vi "MainGui.vi"() -> ()   [LabVIEW 2016]
uses:
  MainGui.TopBar.ctl
  Tools/TouchPanel/TouchPanel.Keyboard.ctl
  Tools/EventLog/EventLog.Gui.Sets.ctl
  Tools/EventLog/EventLog.EventLevelOperatorGui.ctl
  Drivers/PLC/PLC.CheckStatusReassembly.ctl
  MainGui.Action.ctl
  <vilib>/Utility/miscctls.llb/LVRowAndColumnTypeDef.ctl
  <vilib>/Utility/miscctls.llb/LVRowAndColumnUnsignedTypeDef.ctl
  MainGui.UserMsg.ctl
  Tools/Translator/Translator.Message.ctl
  Tools/User/User.Level.ctl
  Tools/CitTemplate/citTemplate.errData.ctl
  Tools/EventLog/EventLog.EventSource.ctl
  Drivers/PLC/PLC.State.ctl
  Database/Database.Gui.ctl
  Database/Database.Gui.SingleTestValue.ctl
  Tools/Translator/Translator.FormatMessage.vi
  Tools/Config/Config.Global.vi
  Global/ApplicationGlobal.vi
  Drivers/PLC/PLC.Global.vi
  Tools/Translator/Translator.Global.vi
  <vilib>/Utility/inputDevices.llb/closeMouse.vi
  Tools/User/User.Global.vi
  Database/Database.Global.vi
panel:
  out "LastPlcRequest":T1
  out "LastRequestedProduct":cluster{"Variant":string, "Serial":string}
  out "RefreshDelay":timestamp
  in  "MainTab":enum32{"Monitor", "Logs"}(tab)
  in  "TESTER":bool
  in  "op30_2":bool caption="OP30_2"
  in  "op40":bool caption="OP40"
  in  "op30_1":bool caption="OP30_1"
  in  "op20":bool caption="OP20"
  in  "op10":bool caption="OP10"
  in  "check":bool
  in  "Serial":string
  in  "RefNum":string
  in  "StatusTable":i32(listbox)=-1
  in  "LogsMode":enum16{"Live", "Arch"}(ring) caption="Mode"
  in  "LogsOptions":T2 caption="Event.Sets" {"Source" items=["All", "Gui", "Cache", "PLC1", "PLC2", "PLC3", "DB", "DB01", "DB02", "DB03", "DB04", "DB05", "DB06", "DB07", "DB08", "DB09", "DB10", "DB11", "DB12", "DB13", "DB14", "DB15", "DB16"]; "Level" items=["ALL", "Debug", "Info", "Warning", "Error"]; "dtm_End" format="%<%.1X\n%x>T"; "dtm_Begin" format="%<%.1X\n%x>T"}
  out "LogsTable":i32(listbox)
  in  "Btn_Exit":bool
  in  "Btin_LogIn":bool
  in  "Btn_Monitor":bool
  in  "TopBar":T4={"_loop"=4, "time"="", "~flag"=bytes[0], "~touchpanel"=FALSE, "ver"="", "~msg"="", "DB"=0, "PLC"=0} {"PLC" items=["OK", "ALL", "PLC01"]; "DB" items=["OK", "ALL", "ST01"]}
  in  "start here":bool
  out "StatusMsg":string
  out "DeviceID":refnum<k1> caption="device ID"
  in  "Btn_ErrConfirm":bool
  out "ErrMsg":i32(listbox)
  in  "Btn_Logs":bool
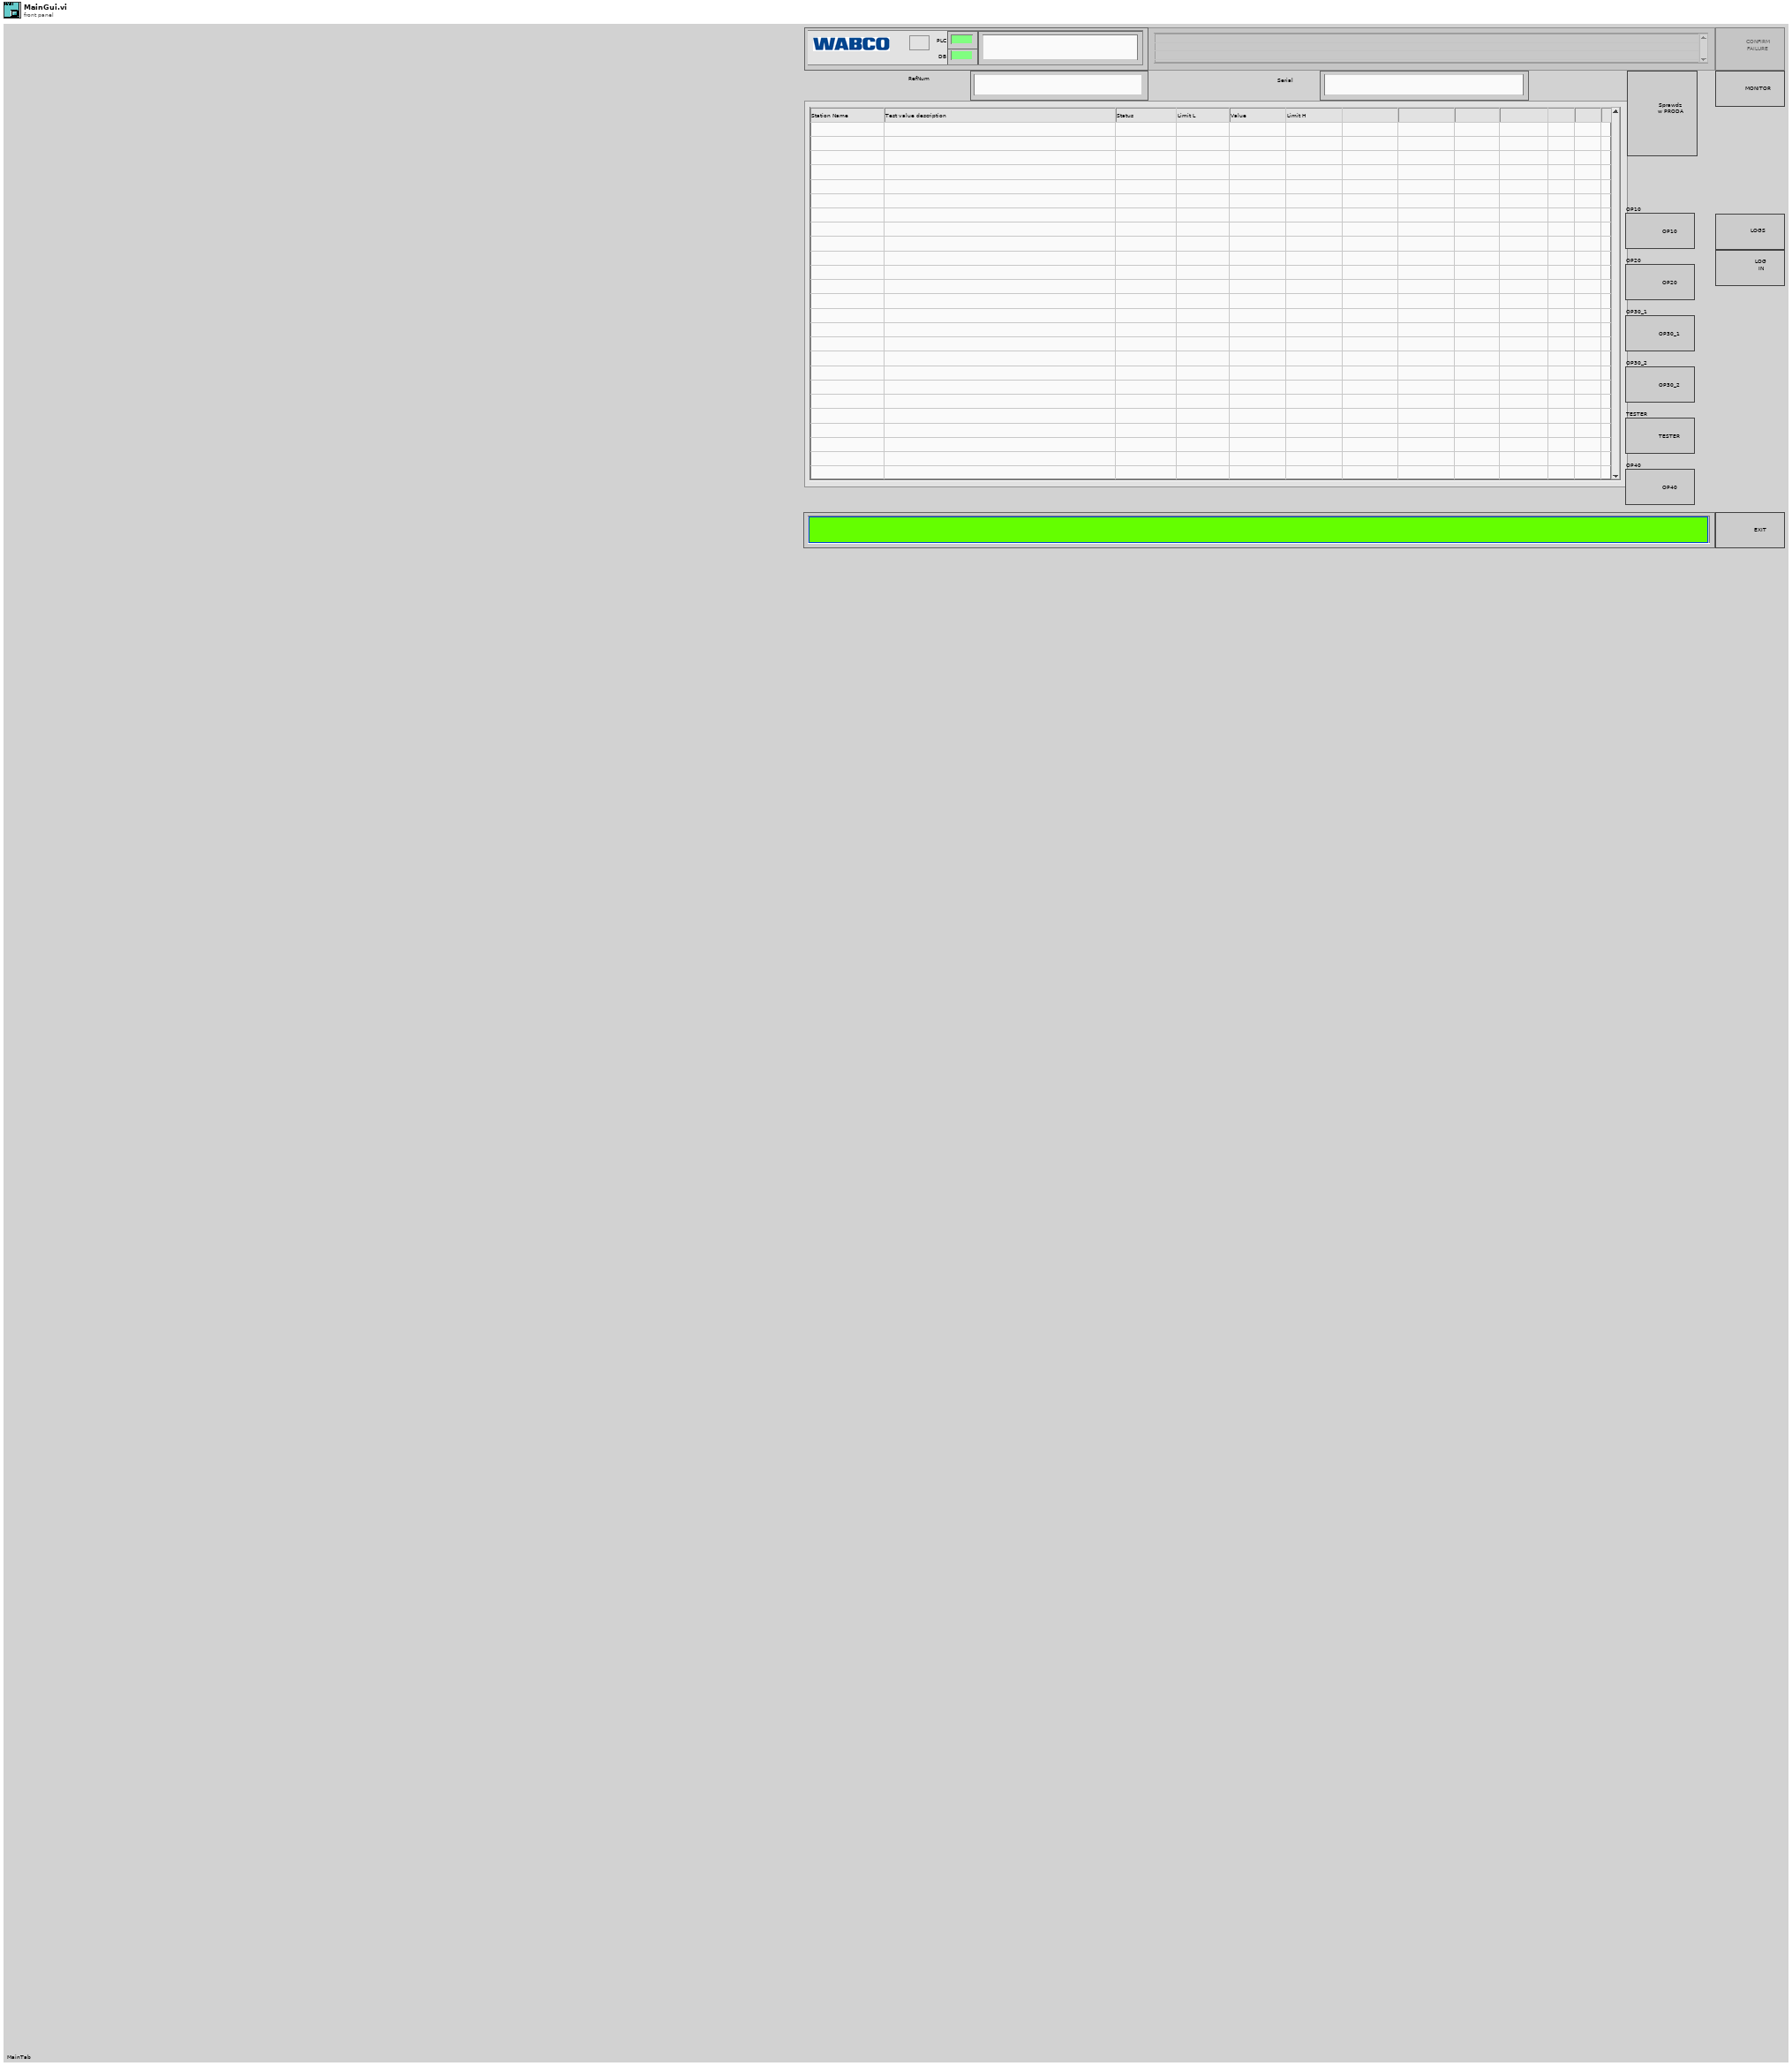
[diagram p1: front panel]
types:
  T1 = typedef "PLC.CheckStatusReassembly.ctl" = cluster{"Ref":string, "Serial":string, "Station":string}
  T2 = typedef "EventLog.Gui.Sets.ctl" = cluster{"IncludeBegin":bool, "dtm_Begin":timestamp, "IncludeEnd":bool, "dtm_End":timestamp, "Events Level Operator":T3, "Level":u16, "Source":u16, "SearchText":string, "Refresh":bool, "Pages":i32, "PageNo":i32, "First":bool, "Prev":bool, "Next":bool, "Last":bool}
  T3 = typedef "EventLog.EventLevelOperatorGui.ctl" = enum16{">=", "=", "<="}
  T4 = typedef "MainGui.TopBar.ctl" = cluster{"_loop":i32, "time":string, "~flag":picture, "~touchpanel":T5, "ver":string, "~msg":string, "DB":u16, "PLC":u16}
  T5 = typedef "TouchPanel.Keyboard.ctl" = bool
  T6 = typedef "Translator.Message.ctl" = enum16{"-", "Event confirmed", "Log out", "Log in", "Shutdown", "Cancel", "Start", "Continue", "Stop", "On", "Off", "OK", "NOK", "NOK %s", "This", "Prev", "Home", "Work", "In progress...", "Missing", "Empty", "Hardware failure", "Initial", "Error %d >> %s", "Error %d >> %s >> %s", "Starting %s", "Quitting %s", "Configured", "Initializing", "Quitting", "Loading", "Running %s", "Stopped", "Summary", "Do you want to continue?", "Do you want to exit?", "Log out?", "System", "All", "IDLE", "Translating...%s", "Not found", "Alarm %s", "Run", "Skip", "Abort", "Repeat", "Please wait...", "Database disconnected", "Login to database successful", "Login to database failed: %d; %s", "Get process step data for %s", "Changeover off", "Changeover into %s", "Product %s | %s found in cache with status %d at previous station", "Product %s | %s found in database with status %d at previous station", "Product %s | %s not found in cache at previous station", "Product %s | %s not found in database at previous station", "Product %s | %s found in cache with status %d at this station (%d repetion)", "Product %s | %s found in database with status %d at this station (%d repetition)", "Product %s | %s not found in cache at this station", "Product %s | %s not found in database at this station", "Product %s | %s found in cache for component %s | %s", "Product %s | %s found in database for component %s | %s", "Product not found in cache for component %s | %s", "Product not found in database for component %s | %s", "Product %s | %s connected with component %s | %s (cache)", "Product %s | %s connected with component %s | %s (database)", "New data for %s | %s (cache)", "New data for %s | %s (database)", "File %s moved (cache)", "File %s deleted (cache)", "Msg %d >> %s", "PLC LifeBit Failure", "Reconnecting DB", "Reconnecting PLC", "Free disk space is below 1GB - contact technician", "Unable to check product status", "Product %s SN %s checked in DB", "Unable To check status from station %s"}
  T7 = enum8{"Enabled", "Disabled", "Disabled and Grayed Out"}
  T8 = typedef "LVRowAndColumnUnsignedTypeDef.ctl" = cluster{"Row":u32, "Column":u32}
  T9 = typedef "LVRowAndColumnTypeDef.ctl" = cluster{"Row":i32, "Column":i32}
  T10 = enum32{"invalid app kind", "Development System", "Run Time System", "Student Edition", "Embedded LabVIEW", "Evaluation", "Custom"}
  T11 = enum32{"Invalid", "Standard", "Closed", "Hidden", "Minimized", "Maximized"}
  T12 = typedef "MainGui.UserMsg.ctl" = cluster{"Msg":T6, "Arguments":variant[], "BgColor":u32, "TxtColor":u32, "Blink":bool}
  T13 = typedef "User.Level.ctl" = enum16{"-", "Operator", "Technician", "Administrator"}
  T14 = typedef "citTemplate.errData.ctl" = cluster{"ts":timestamp, "src":T15, "instance":i32, "action":string, "error":errorcluster, "unconfirmed":bool}
  T15 = typedef "EventLog.EventSource.ctl" = enum16{"All", "Gui", "Cache", "PLC1", "PLC2", "PLC3", "DB", "DB01", "DB02", "DB03", "DB04", "DB05", "DB06", "DB07", "DB08", "DB09", "DB10", "DB11", "DB12", "DB13", "DB14", "DB15", "DB16"}
  T16 = typedef "PLC.State.ctl" = enum32{"Off", "Error", "Idle", "Run"}
  T17 = typedef "Database.Gui.ctl" = cluster{"Station":string, "ButtonEnabled":bool, "Values":T18[]}
  T18 = typedef "Database.Gui.SingleTestValue.ctl" = cluster{"EV_name":string, "Value":dbl, "LimitL":dbl, "LimitH":dbl, "Status":u8}
  T19 = typedef "MainGui.Action.ctl" = enum32{"idle", "constructor", "destructor", "--- MainGui ---", "Gui.Translate", "Error.Update", "Error.Confirm", "TopBar.Update", "Buttons.Update", "StatusMsg.Update", "StatusTable.Update", "LogsTable.Update", "PLCReasemblyDone"}
  T20 = typedef "LVPositionTypeDef.ctl" = cluster{"Left":i32, "Top":i32}
  T21 = typedef "PLC.Data.Status.ctl" = cluster{"Idx":i32, "ConnRef":u64, "State":T16, "LiveBitTimer":timestamp}
  T22 = typedef "Database.Handler.Data.Status.ctl" = cluster{"Run":bool, "Handle":i32, "ConnTS":timestamp, "DbTime":timestamp, "DbTimeOffset":dbl}
  T23 = typedef "Database.Data.Sets.ctl" = cluster{"Enable":bool, "ConnString":string, "SystemName":string, "Process.Begin":bool, "Process.End":bool}
  T24 = typedef "PLC.Data.Sets.ctl" = cluster{"Enable":bool, "IP":string, "Rack":i32, "Slot":i32, "LifeBitTimer_s":dbl, "DataBlockAddr_PCStatus":i32, "DataBlockAddr_PLCStatus":i32, "DataBlockAddr_PLCNewData":i32[], "DataBlockSize_PLCNewData":i32[], "DataBlockAddr_PLCChangeOver":i32[], "DataBlockSize_PLCChangeOver":i32[], "DataBlockAddr_PCChangeOver":i32[], "DataBlockAddr_PLCCheckStatus":i32[], "DataBlockSize_PLCCheckStatus":i32[], "DataBlockAddr_PCCheckStatus":i32[]}
  T25 = typedef "EventLog.EventGui.ctl" = cluster{"ts":dbl, "lev":T26, "src":T15, "msg":T6, "arg":variant[], "msg_str":string}
  T26 = typedef "EventLog.EventLevel.ctl" = enum8{"Debug", "Info", "Warning", "Error"}
  T27 = cluster{"Ref":bool, "Serial":bool, "Station":bool}
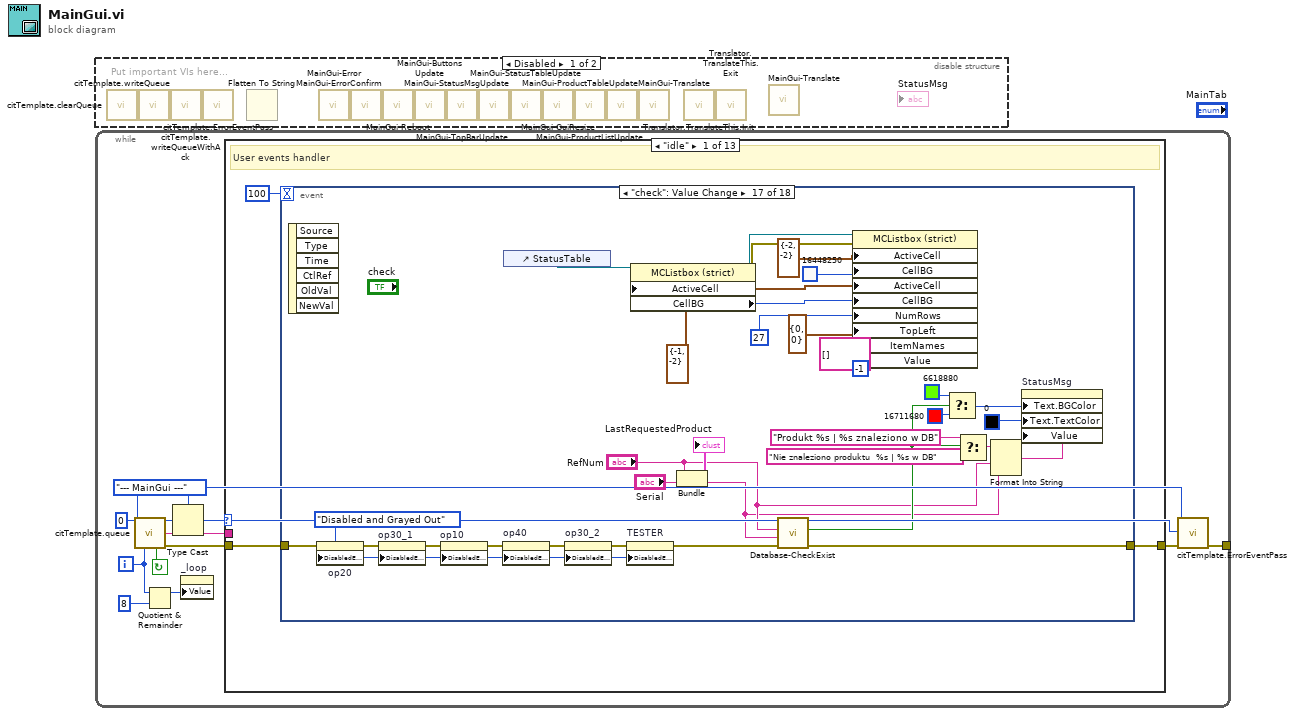
[diagram p0: block diagram]
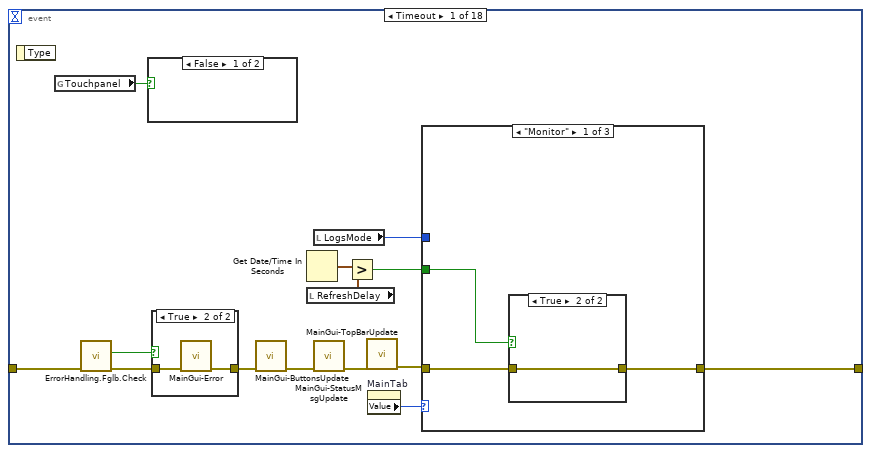
[diagram p3: hidden frame]
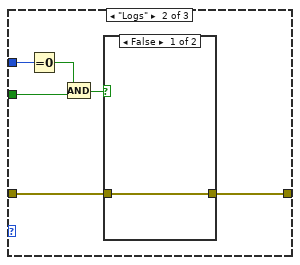
[diagram p6: hidden frame]
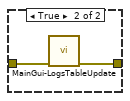
[diagram p7: hidden frame]
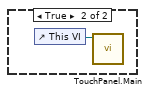
[diagram p9: hidden frame]
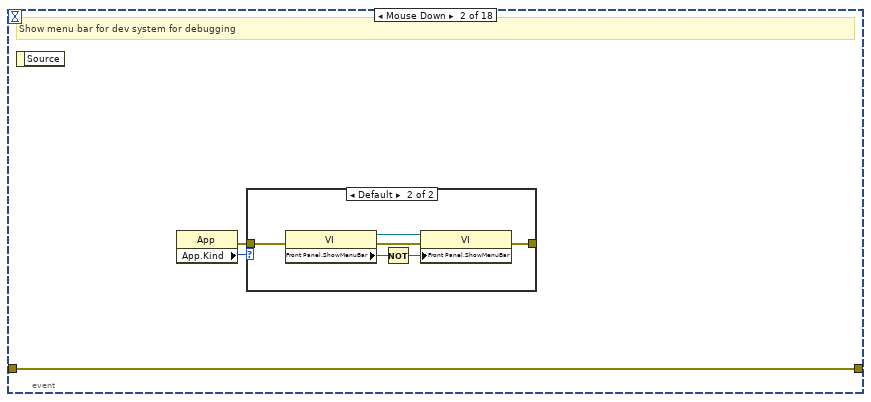
[diagram p10: hidden frame]
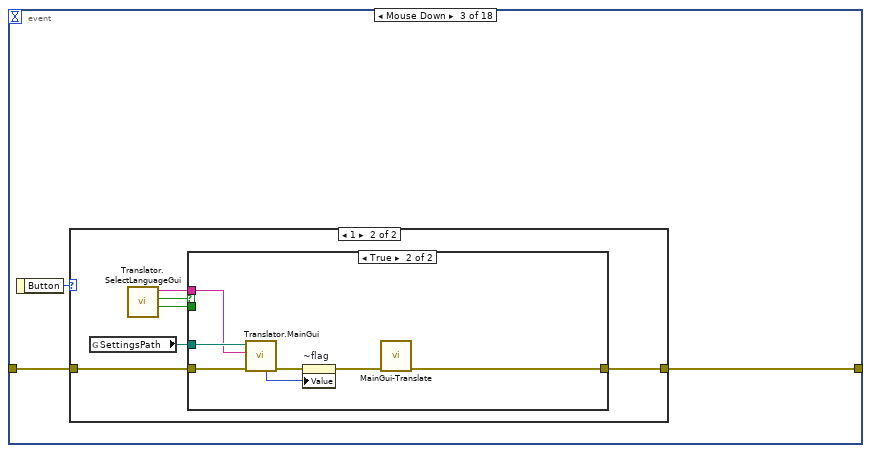
[diagram p12: hidden frame]
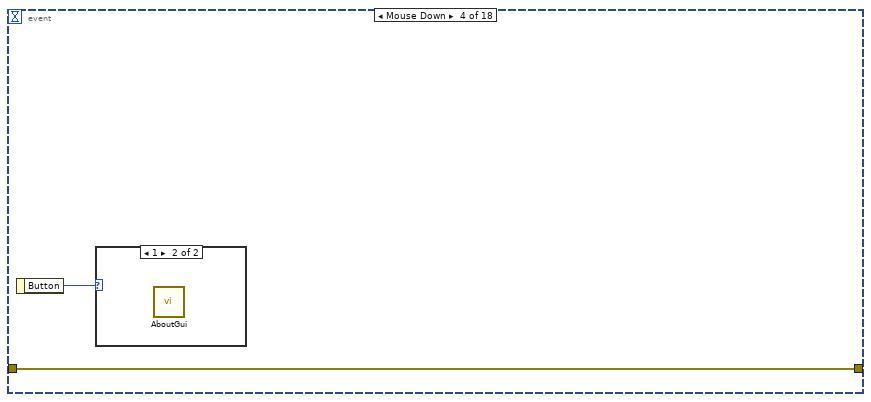
[diagram p15: hidden frame]
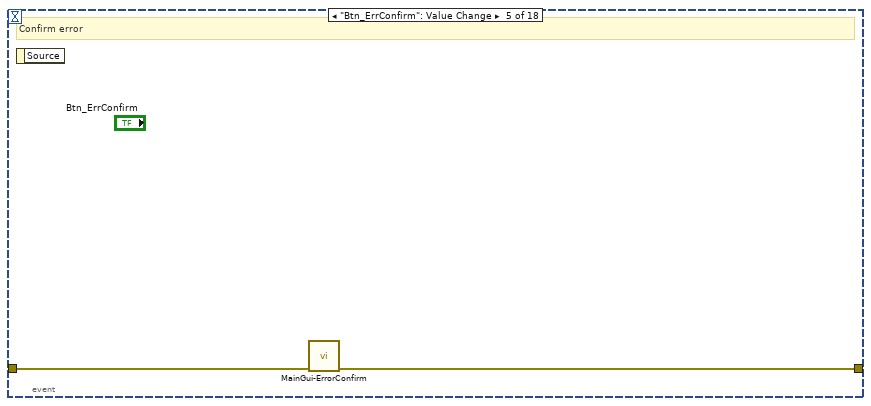
[diagram p17: hidden frame]
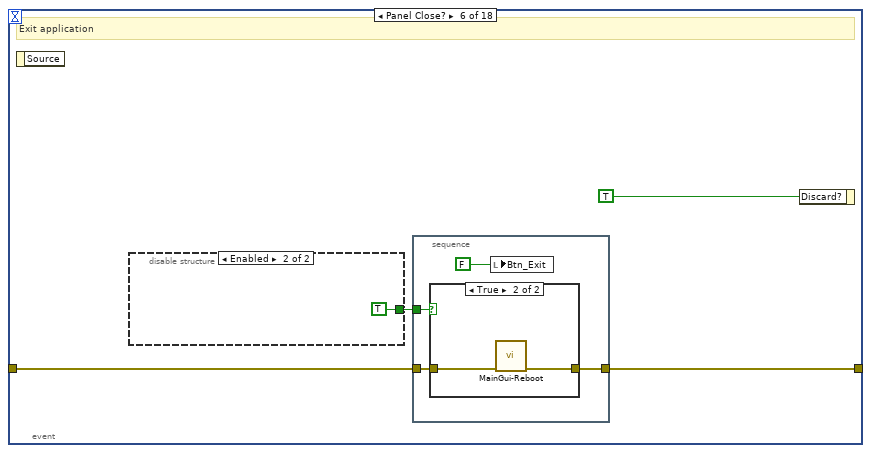
[diagram p18: hidden frame]
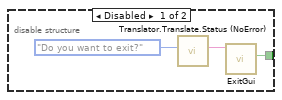
[diagram p19: hidden frame]
diagram:
  n1 = disable-structure shown="Disabled" {
    frame Disabled {
      # "Put important VIs here..."
      n2 = call "citTemplate.clearQueue.vi"() -> ()  [unwired: 14 in, 2 out]
      n3 = call "citTemplate.writeQueue.vi"() -> ()  [unwired: 15 in, 1 out]
      n4 = call "citTemplate.writeQueueWithAck.vi"() -> ()  [unwired: 13 in, 3 out]
      n5 = call "citTemplate.ErrorEventPass.vi"() -> ()  [unwired: 11 in, 1 out]
      n6 = Flatten To String() -> ()  [unwired: 4 in, 3 out]
      n7 = call "MainGui-Error.vi"() -> ()  [unwired: 11 in, 1 out]
      n8 = call "MainGui-ErrorConfirm.vi"() -> ()  [unwired: 11 in, 1 out]
      n9 = call "MainGui-Reboot.vi"() -> ()  [unwired: 11 in, 1 out]
      n10 = call "MainGui-ButtonsUpdate.vi"() -> ()  [unwired: 11 in, 1 out]
      n11 = call "MainGui-TopBarUpdate.vi"() -> ()  [unwired: 11 in, 1 out]
      n12 = call "MainGui-StatusMsgUpdate.vi"() -> ()  [unwired: 11 in, 1 out]
      n13 = call "MainGui-StatusTableUpdate.vi"() -> ()  [unwired: 11 in, 1 out]
      n14 = call "MainGui-GuiResize.vi"() -> ()  [unwired: 11 in, 1 out]
      n15 = call "MainGui-ProductListUpdate.vi"() -> ()  [unwired: 11 in, 1 out]
      n16 = call "MainGui-ProductTableUpdate.vi"() -> ()  [unwired: 11 in, 1 out]
      n17 = call "MainGui-Translate.vi"() -> ()  [unwired: 11 in, 1 out]
      n18 = call "Translator.TranslateThis.Init.vi"() -> ()  [unwired: 11 in, 1 out]
      n19 = call "Translator.TranslateThis.Exit.vi"() -> ()  [unwired: 11 in, 1 out]
      n20 = call "MainGui-Translate.vi"() -> ()  [unwired: 11 in, 1 out]
    }
    frame Enabled {
    }
  }
  n21 = while {
    tunnel: [w5] -> _
    i -> [w6]
    stop <- w9 continue-if-true
    w8 = MainGui.Action."--- MainGui ---" ("Action")
    n22 = call "citTemplate.queue.vi"("ms timeout (250 ms)"=0, "event enum"=w8, "iteration (-1)"=w6) -> ("event out"=w12:u32, "(flatten) data out"=w11:string, "continue"=w9:bool, "error out"=w10:errorcluster)  [unwired: 2 in, 7 out]
    n23 = Quotient & Remainder(x=w6, y=8) -> (x-y*floor(x/y)=w1:i32)  [unwired: 1 out]
    n24 = Type Cast(type=w8, x=w12) -> (*(type *) &x=w4:T19)
    n25 = property on="_loop" class="Ring (strict)"("Value"=w1) -> ()  [unwired: 2 in, 2 out]
    n26 = case shown="\"idle\"" w4 {
      tunnel: w11 -> [_ _ _ w315 _ _ _ _ _ _ w458 _ w568]
      tunnel: w10 -> [w15 w228 w285 w317 w319 w323 w360 w361 w409 w413 w460 w517 w587]
      tunnel: [w14 w227 w284 w314 w322 w324 w359 w361 w409 w412 w445 w516 w569] -> w2
      frame "idle" {
        # "User events handler"
        n27 = event shown="[16] \"check\": Value Change" {
          selector: _ -> [_ _ _ _ _ _ _ _ _ _ _ _ _ _ _ _ _ _]
          dyn-events: _ -> [_ _ _ _ _ _ _ _ _ _ _ _ _ _ _ _ _ _]
          timeout: 100 -> [_ _ _ _ _ _ _ _ _ _ _ _ _ _ _ _ _ _]
          tunnel: w15 -> [w25 w51 w60 w77 w80 w83 w98 w113 w119 w125 w128 w135 w140 w148 w156 w161 w180 w220]
          tunnel: [w26 w51 w59 w77 w79 w82 w97 w113 w119 w125 w127 w134 w140 w148 w156 w161 w193 w208] -> w14
          event Timeout {
            n28 = event-data() -> ()  [unwired: 1 in, 1 out]
            n29 = global read "Config.Global.vi" "Touchpanel"() -> (w29:bool)
            n30 = call "ErrorHandling.Fglb.Check.vi"("error in (no error)"=w25) -> ("error out"=w24:errorcluster, "changed?"=w23:bool)  [unwired: 9 in]
            n31 = case shown="False" w29 {
              frame False {
              }
              frame True {
                n32 = control-ref of="This VI"() -> (w48:refnum<vi>)
                n33 = call "TouchPanel.Main.vi"("VI ref"=w48) -> ()  [unwired: 9 in, 2 out]
              }
            }
            n34 = case shown="True" w23 {
              tunnel: [w30 w32] -> w28
              tunnel: w24 -> [w30 w31]
              frame False {
              }
              frame True {
                n35 = call "MainGui-Error.vi"("error in (no error)"=w31) -> ("error out"=w32:errorcluster)  [unwired: 10 in]
              }
            }
            n36 = call "MainGui-ButtonsUpdate.vi"("error in (no error)"=w28) -> ("error out"=w18:errorcluster)  [unwired: 10 in]
            n37 = Get Date/Time In Seconds() -> (seconds since 1Jan1904=w22:timestamp)
            n38 = local read "RefreshDelay"() -> (w21:timestamp)
            n39 = local read "LogsMode"() -> (w19:enum16{"Live", "Arch"})
            n40 = call "MainGui-StatusMsgUpdate.vi"("error in (no error)"=w18) -> ("error out"=w17:errorcluster)  [unwired: 10 in]
            n41 = Greater?(x=w22, y=w21) -> (0:w20:bool)
            n42 = call "MainGui-TopBarUpdate.vi"("error in (no error)"=w17) -> ("error out"=w16:errorcluster)  [unwired: 10 in]
            n43 = property on="MainTab" class="TabCtl (strict)"() -> ("Value"=w27:enum32{"Monitor", "Logs"})  [unwired: 2 in, 2 out]
            n44 = case shown="\"Monitor\"" w27 {
              tunnel: w16 -> [w35 w39 w47]
              tunnel: [w34 w38 w47] -> w26
              tunnel: w20 -> [w33 w42 _]
              tunnel: w19 -> [_ w43 _]
              frame "Monitor" {
                n45 = case shown="True" w33 {
                  tunnel: w35 -> [w36 w37]
                  tunnel: [w36 w37] -> w34
                  frame False {
                  }
                  frame True {
                  }
                }
              }
              frame "Logs" {
                n46 = Equal To 0?(x=w43) -> (x = 0?=w41:bool)
                n47 = Compound Arithmetic op=AND(w41, w42) -> (w40:bool)
                n48 = case shown="False" w40 {
                  tunnel: w39 -> [w44 w46]
                  tunnel: [w44 w45] -> w38
                  frame False {
                  }
                  frame True {
                    n49 = call "MainGui-LogsTableUpdate.vi"("error in (no error)"=w46) -> ("error out"=w45:errorcluster)  [unwired: 10 in]
                  }
                }
              }
              frame Default {
              }
            }
          }
          event Mouse Down {
            # "Show menu bar for dev system for debugging"
            n50 = event-data() -> ()  [unwired: 1 in, 1 out]
            n51 = property class="App"() -> (error out=w49:errorcluster, "App.Kind"=w50:T10)  [unwired: 2 in, 1 out]
            n52 = case shown="Default" w50 {
              tunnel: w49 -> [w52 w54]
              tunnel: [w52 w53] -> _
              frame "Run Time System" {
              }
              frame Default {
                n53 = property class="VI"(error in=w54) -> (reference out=w58:refnum<vi>, error out=w57:errorcluster, "Front Panel.ShowMenuBar"=w56:bool)  [unwired: 1 in]
                n54 = Not(x=w56) -> (.not. x?=w55:bool)
                n55 = property class="VI"(reference=w58, error in=w57, "Front Panel.ShowMenuBar"=w55) -> (error out=w53:errorcluster)  [unwired: 1 out]
              }
            }
          }
          event Mouse Down {
            n56 = event-data() -> ("Button"=w61:u16)  [unwired: 1 in]
            n57 = case shown="1" w61 {
              tunnel: w60 -> [w62 w66]
              tunnel: [w62 w65] -> w59
              frame Default {
              }
              frame 1 {
                n58 = global read "ApplicationGlobal.vi" "SettingsPath"() -> (w63:path)
                n59 = call "Translator.SelectLanguageGui.vi"() -> ("english"=w67:bool, "changed"=w68:bool, "Language"=w64:string)  [unwired: 9 in]
                n60 = case shown="True" w68 {
                  tunnel: w67 -> [_ _]
                  tunnel: w66 -> [w69 w76]
                  tunnel: [w69 w70] -> w65
                  tunnel: w64 -> [_ w74]
                  tunnel: w63 -> [_ w75]
                  frame False {
                  }
                  frame True {
                    n61 = call "Translator.MainGui.vi"("~error in"=w76, "~Language in use"=w74, "~Translation folder"=w75) -> ("~error out"=w73:errorcluster, "~flag small"=w72:picture)  [unwired: 5 in, 2 out]
                    n62 = property on="~flag" class="Pict"(error in=w73, "Value"=w72) -> (error out=w71:errorcluster)  [unwired: 1 in, 1 out]
                    n63 = call "MainGui-Translate.vi"("error in (no error)"=w71) -> ("error out"=w70:errorcluster)  [unwired: 10 in]
                  }
                }
              }
            }
          }
          event Mouse Down {
            n64 = event-data() -> ("Button"=w78:u16)  [unwired: 1 in]
            n65 = case shown="1" w78 {
              frame Default {
              }
              frame 1 {
                n66 = call "AboutGui.vi"() -> ()  [unwired: 12 in]
              }
            }
          }
          event "Btn_ErrConfirm": Value Change {
            # "Confirm error"
            n67 = event-data() -> ()  [unwired: 1 in, 1 out]
            n68 = call "MainGui-ErrorConfirm.vi"("error in (no error)"=w80) -> ("error out"=w79:errorcluster)  [unwired: 10 in]
          }
          event Panel Close? {
            # "Exit application"
            n69 = event-data() -> ()  [unwired: 1 in, 1 out]
            n70 = disable-structure shown="Enabled" {
              disable-tunnel: [w87 TRUE ("ok")] -> w84
              frame Disabled {
                n71 = call "Translator.Translate.Status (NoError).vi"("msg"=Translator.Message."Do you want to exit?") -> ("Translated Msg"=w85:string)  [unwired: 10 in]
                n72 = call "ExitGui.vi"("Message"=w85) -> ("ok"=w87:bool)  [unwired: 9 in, 1 out]
              }
              frame Enabled {
              }
            }
            n73 = stacked-sequence {
              tunnel: [w92] -> w82
              tunnel: w83 -> [w90]
              tunnel: w84 -> [w89]
              frame #0 {
                n74 = case shown="True" w89 {
                  tunnel: w90 -> [w93 w94]
                  tunnel: [w93 w95] -> w92
                  frame False {
                  }
                  frame True {
                    n75 = call "MainGui-Reboot.vi"("error in (no error)"=w94) -> ("error out"=w95:errorcluster)  [unwired: 10 in]
                  }
                }
                n76 = local write "Btn_Exit"(FALSE ("Btn_SelMode")) -> ()
              }
            }
            n77 = event-data("Discard?"=TRUE) -> ()  [unwired: 1 in, 1 out]
          }
          event "Btn_Exit": Value Change {
            # "Exit application"
            n78 = event-data() -> ()  [unwired: 1 in, 1 out]
            n79 = disable-structure shown="Disabled" {
              disable-tunnel: [w102 TRUE ("ok")] -> w99
              frame Disabled {
                n80 = call "Translator.Translate.Status (NoError).vi"("msg"=Translator.Message."Do you want to exit?") -> ("Translated Msg"=w100:string)  [unwired: 10 in]
                n81 = call "ExitGui.vi"("Message"=w100) -> ("ok"=w102:bool)  [unwired: 9 in, 1 out]
              }
              frame Enabled {
              }
            }
            n82 = property on="Btn_Exit" class="Bool (strict)"("Value"=FALSE ("Btn_Exit")) -> ()  [unwired: 2 in, 2 out]
            n83 = stacked-sequence {
              tunnel: [w106] -> w97
              tunnel: w98 -> [w105]
              tunnel: w99 -> [w104]
              frame #0 {
                n84 = case shown="True" w104 {
                  tunnel: w105 -> [w107 w108]
                  tunnel: [w107 w109] -> w106
                  frame False {
                  }
                  frame True {
                    n85 = call "MainGui-Reboot.vi"("error in (no error)"=w108) -> ("error out"=w109:errorcluster)  [unwired: 10 in]
                  }
                }
              }
            }
          }
          event "Btin_LogIn": Value Change {
            # "Log in/out"
            n86 = event-data() -> ()  [unwired: 1 in, 1 out]
            n87 = global write "ApplicationGlobal.vi" "Unlock"("Btin_LogIn") -> ()
            n88 = Select(t=T7."Enabled" ("Disabled"), s="Btin_LogIn", f=T7."Disabled and Grayed Out") -> ()  [unwired: 1 out]
          }
          event "Btn_Monitor": Value Change {
            w118 = TRUE ("Btn_Monitor")
            n89 = event-data() -> ()  [unwired: 1 in, 1 out]
            n90 = property on="MainTab" class="TabCtl (strict)"("Value"=0) -> ()  [unwired: 2 in, 2 out]
            n91 = property on="Btn_Monitor" class="Bool (strict)"("Value"=w118) -> (error out=w114:errorcluster)  [unwired: 2 in, 1 out]
            n92 = Not(x=w118) -> (.not. x?=w116:bool)
            n93 = Get Date/Time In Seconds() -> (seconds since 1Jan1904=w115:timestamp)
            n94 = local write "RefreshDelay"(w115) -> ()
            n95 = property on="Btn_Logs" class="Bool (strict)"(error in=w114, "Value"=w116) -> ()  [unwired: 1 in, 2 out]
          }
          event "Btn_Logs": Value Change {
            w124 = TRUE ("Btn_Monitor")
            n96 = event-data() -> ()  [unwired: 1 in, 1 out]
            n97 = property on="MainTab" class="TabCtl (strict)"("Value"=1) -> ()  [unwired: 2 in, 2 out]
            n98 = property on="Btn_Logs" class="Bool (strict)"("Value"=w124) -> (error out=w123:errorcluster)  [unwired: 2 in, 1 out]
            n99 = Not(x=w124) -> (.not. x?=w121:bool)
            n100 = property on="Btn_Monitor" class="Bool (strict)"(error in=w123, "Value"=w121) -> ()  [unwired: 1 in, 2 out]
            n101 = Get Date/Time In Seconds() -> (seconds since 1Jan1904=w120:timestamp)
            n102 = local write "RefreshDelay"(w120) -> ()
          }
          event "LogsMode": Value Change {
            n103 = event-data() -> ()  [unwired: 1 in, 1 out]
            n104 = Greater Than 0?(x="LogsMode") -> (x > 0?=w130:bool)
            n105 = Select(t=T7."Enabled" ("Disabled"), s=w130, f=T7."Disabled" ("Disabled")) -> (s? t:f=w126:T7)
            n106 = Not(x=w130) -> (.not. x?=w129:bool)
            n107 = property on="PageNo" class="DigNum (strict)"("DisabledEnum"=w126) -> ()  [unwired: 2 in, 2 out]
            n108 = property on="LogsTable" class="MCListbox (strict)"("HScrollVis"=w129) -> ()  [unwired: 2 in, 2 out]
            n109 = property on="First" class="Bool (strict)"("DisabledEnum"=w126) -> ()  [unwired: 2 in, 2 out]
            n110 = property on="Prev" class="Bool (strict)"("DisabledEnum"=w126) -> ()  [unwired: 2 in, 2 out]
            n111 = call "MainGui-LogsTableUpdate.vi"("error in (no error)"=w128) -> ("error out"=w127:errorcluster)  [unwired: 10 in]
            n112 = property on="Next" class="Bool (strict)"("DisabledEnum"=w126) -> ()  [unwired: 2 in, 2 out]
            n113 = property on="Last" class="Bool (strict)"("DisabledEnum"=w126) -> ()  [unwired: 2 in, 2 out]
          }
          event Value Change {
            n114 = event-data() -> ()  [unwired: 1 in, 1 out]
            n115 = call "MainGui-LogsTableUpdate.vi"("error in (no error)"=w135) -> ("error out"=w134:errorcluster)  [unwired: 10 in]
          }
          event Value Change {
            n116 = event-data() -> ()  [unwired: 1 in, 1 out]
            n117 = local read "LogsOptions"() -> (w139:T2)
            n118 = Bundle By Name(cluster=w139, "PageNo"=0, "First"=FALSE) -> (w138:T2)
            n119 = local write "LogsOptions"(w138) -> ()
          }
          event Value Change {
            n120 = event-data() -> ()  [unwired: 1 in, 1 out]
            n121 = local read "LogsOptions"() -> (w146:T2)
            n122 = Unbundle By Name(w146) -> ("PageNo"=w143:i32)
            n123 = Decrement(x=w143) -> (x-1=w145:i32)
            n124 = Max & Min(x=w145, y=i64 0 ("Value (Signaling)")) -> (max(x,y)=w142:i64)  [unwired: 1 out]
            n125 = Bundle By Name(cluster=w146, "PageNo"=w142, "Prev"=FALSE ("First")) -> (w147:T2)
            n126 = local write "LogsOptions"(w147) -> ()
          }
          event Value Change {
            n127 = event-data() -> ()  [unwired: 1 in, 1 out]
            n128 = local read "LogsOptions"() -> (w154:T2)
            n129 = Unbundle By Name(w154) -> ("PageNo"=w152:i32, "Pages"=w151:i32)
            n130 = Increment(x=w152) -> (x+1=w153:i32)
            n131 = Max & Min(x=w153, y=w151) -> (min(x,y)=w149:i32)  [unwired: 1 out]
            n132 = Bundle By Name(cluster=w154, "PageNo"=w149, "Next"=FALSE ("First")) -> (w155:T2)
            n133 = local write "LogsOptions"(w155) -> ()
          }
          event Value Change {
            n134 = event-data() -> ()  [unwired: 1 in, 1 out]
            n135 = local read "LogsOptions"() -> (w159:T2)
            n136 = Unbundle By Name(w159) -> ("Pages"=w158:i32)
            n137 = Bundle By Name(cluster=w159, "PageNo"=w158, "Last"=FALSE) -> (w160:T2)
            n138 = local write "LogsOptions"(w160) -> ()
          }
          event "check": Value Change {
            w181 = T7."Disabled and Grayed Out" ("Disabled")
            w189 = T9 {"Row"=-1, "Column"=-2} ("Active Cell:Active Cell")
            n139 = event-data() -> ()  [unwired: 1 in, 6 out]
            n140 = property on="op20" class="Bool"(error in=w180, "DisabledEnum"=w181) -> (error out=w179:errorcluster)  [unwired: 1 in, 1 out]
            n141 = property on="op30_1" class="Bool"(error in=w179, "DisabledEnum"=w181) -> (error out=w178:errorcluster)  [unwired: 1 in, 1 out]
            n142 = property on="op10" class="Bool"(error in=w178, "DisabledEnum"=w181) -> (error out=w177:errorcluster)  [unwired: 1 in, 1 out]
            n143 = property on="op40" class="Bool"(error in=w177, "DisabledEnum"=w181) -> (error out=w176:errorcluster)  [unwired: 1 in, 1 out]
            n144 = control-ref of="StatusTable"() -> (w182:refnum<vi>)
            n145 = property on="op30_2" class="Bool"(error in=w176, "DisabledEnum"=w181) -> (error out=w175:errorcluster)  [unwired: 1 in, 1 out]
            n146 = property on="TESTER" class="Bool"(error in=w175, "DisabledEnum"=w181) -> (error out=w174:errorcluster)  [unwired: 1 in, 1 out]
            n147 = property on="Property Node" class="MCListbox (strict)"(reference=w182, "ActiveCell"=w189) -> (reference out=w173:refnum<vi>, error out=w187:errorcluster, "CellBG"=w188:u32)  [unwired: 1 in]
            n148 = Bundle("RefNum"="RefNum", "Serial"="Serial") -> (→"LastRequestedProduct":cluster{"RefNum":string, "Serial":string})  [unwired: 1 in]
            n149 = call "Database-CheckExist.vi"("error in"=w174, "Serial"="Serial", "Ref"="RefNum") -> ("error out"=w193:errorcluster, "Found"=w164:bool)  [unwired: 7 in]
            n150 = property on="Property Node" class="MCListbox (strict)"(reference=w173, error in=w187, "ActiveCell"=T9 {"Row"=-2, "Column"=-2} ("Active Cell:Active Cell"), "CellBG"=u32 16448250, "ActiveCell"=w189, "CellBG"=w188, "NumRows"=27, "TopLeft"=T8 {"Row"=0, "Column"=0} ("Top Left Visible Cell"), "ItemNames"=string[][] [] ("Item Names"), "Value"=-1 ("StatusTable")) -> ()  [unwired: 2 out]
            n151 = Select(t=u32 6618880, s=w164, f=u32 16711680) -> (s? t:f=w165:u32)
            n152 = Select(t="Produkt %s | %s znaleziono w DB", s=w164, f="Nie znaleziono produktu  %s | %s w DB") -> (s? t:f=w170:string)
            n153 = Format Into String(format string=w170, "RefNum", "Serial") -> (resulting string=w169:string)  [unwired: 2 in, 1 out]
            n154 = property on="StatusMsg" class="Str"("Text.BGColor"=w165, "Text.TextColor"=u32 0, "Value"=w169) -> ()  [unwired: 2 in, 2 out]
          }
          event "op10", "op20", "op30_1", "op40", "op30_2", "TESTER": Value Change {
            w194 = T7."Disabled and Grayed Out" ("Disabled")
            w217 = T9 {"Row"=-1, "Column"=-2} ("Active Cell:Active Cell")
            n155 = event-data() -> ("CtlRef"=w222:refnum<vi>)  [unwired: 1 in]
            n156 = local read "LastRequestedProduct"() -> (w225:cluster{"Variant":string, "Serial":string})
            n157 = property on="op20" class="Bool"("DisabledEnum"=w194) -> (error out=w201:errorcluster)  [unwired: 2 in, 1 out]
            n158 = property class="Bool"(reference=w222) -> ("Caption.Text"=w221:string)  [unwired: 1 in, 2 out]
            n159 = property on="op30_1" class="Bool"(error in=w201, "DisabledEnum"=w194) -> (error out=w200:errorcluster)  [unwired: 1 in, 1 out]
            n160 = Unbundle By Name(w225) -> ("Variant"=w224:string, "Serial"=w223:string)
            n161 = property on="op10" class="Bool"(error in=w200, "DisabledEnum"=w194) -> (error out=w199:errorcluster)  [unwired: 1 in, 1 out]
            n162 = Bundle By Name(cluster=T1 {"Ref"="", "Serial"="", "Station"=""} ("Cluster"), "Ref"=w224, "Serial"=w223, "Station"=w221) -> (w202:T1)
            "LastPlcRequest" <- w202
            n163 = property on="op40" class="Bool"(error in=w199, "DisabledEnum"=w194) -> (error out=w198:errorcluster)  [unwired: 1 in, 1 out]
            n164 = call "PLC-Reasembly.vi"("error in"=w220, "Reasembly data"=w202) -> ("error out"=w208:errorcluster)  [unwired: 9 in]
            n165 = property on="op30_2" class="Bool"(error in=w198, "DisabledEnum"=w194) -> (error out=w197:errorcluster)  [unwired: 1 in, 1 out]
            n166 = Unbundle By Name(w202) -> ("Ref"=w207:string, "Serial"=w206:string, "Station"=w205:string)
            n167 = control-ref of="StatusTable"() -> (w210:refnum<vi>)
            n168 = property on="TESTER" class="Bool"(error in=w197, "DisabledEnum"=w194) -> ()  [unwired: 1 in, 2 out]
            n169 = property on="check" class="Bool"("DisabledEnum"=w194) -> ()  [unwired: 2 in, 2 out]
            n170 = property on="Property Node" class="MCListbox (strict)"(reference=w210, "ActiveCell"=w217) -> (reference out=w209:refnum<vi>, error out=w215:errorcluster, "CellBG"=w216:u32)  [unwired: 1 in]
            n171 = Format Into String(initial string="Oczekiwanie na potwierdzenie %s | %s ze stacji %s", w207, w206, w205) -> (resulting string=w204:string)  [unwired: 2 in, 1 out]
            n172 = property on="StatusMsg" class="Str"("Text.BGColor"=u32 16761760, "Text.TextColor"=u32 0, "Value"=w204) -> ()  [unwired: 2 in, 2 out]
            n173 = property on="Property Node" class="MCListbox (strict)"(reference=w209, error in=w215, "ActiveCell"=T9 {"Row"=-2, "Column"=-2} ("Active Cell:Active Cell"), "CellBG"=u32 16448250, "ActiveCell"=w217, "CellBG"=w216, "NumRows"=27, "TopLeft"=T8 {"Row"=0, "Column"=0} ("Top Left Visible Cell"), "ItemNames"=string[][] [] ("Item Names"), "Value"=-1 ("StatusTable")) -> ()  [unwired: 2 out]
          }
        }
      }
      frame "constructor" {
        # "Application initialization actions"
        n174 = stacked-sequence {
          tunnel: w228 -> [_ _ _ _ _ _ w277]
          tunnel: [_ _ _ _ _ _ w277] -> w227
          frame #0 {
            # "Init FP"
            n175 = property class="App"() -> ("App.Kind"=w233:T10)  [unwired: 2 in, 2 out]
            n176 = property on="TopBar" class="Clust (strict)"() -> (error out=w237:errorcluster, "Position"=w236:T20)  [unwired: 2 in, 1 out]
            n177 = Not Equal?(x=w233, y=T10."Run Time System") -> (x != y?=w231:bool)
            n178 = global write "ApplicationGlobal.vi" "Unlock"(w231) -> ()
            n179 = property on="Pane" class="Pane"(error in=w237, "Origin"=w236) -> (error out=w234:errorcluster)  [unwired: 1 in, 1 out]
            n180 = property class="VI"(error in=w234, "Front Panel.ShowMenuBar"=FALSE ("Front Panel Window:Show Menu Bar"), "Front Panel.TitleBarVis"=TRUE ("Front Panel Window:Title Bar Visible"), "FP.State"=T11."Maximized" ("Front Panel Window:State")) -> ()  [unwired: 1 in, 2 out]
          }
          frame #1 {
            # "Open references"
            n181 = call <vilib>:"Initialize Mouse.vi"() -> ("device ID"=→"DeviceID":refnum<k1>)  [unwired: 10 in, 1 out]
          }
          frame #2 {
            n182 = global read "PLC.Global.vi" "PLC1.Status"() -> (w251:T21)
            n183 = Build Array(w251) -> (w250:T21[])
            n184 = for {
              tunnel: w250 -> [_] mode=indexing
              tunnel: [w257] -> w249 mode=indexing
              i -> [w259]
              n185 = Increment(x=w259) -> (x+1=w256:i32)
              n186 = Format Into String(format string="PLC%02d", w256) -> (resulting string=w257:string)  [unwired: 2 in, 1 out]
            }
            n187 = for {
              N: 1 -> [_]
              tunnel: [w253] -> w240 mode=indexing
              i -> [w255]
              n188 = Increment(x=w255) -> (x+1=w252:i32)
              n189 = Format Into String(format string="ST%02d", w252) -> (resulting string=w253:string)  [unwired: 2 in, 1 out]
            }
            n190 = Build Array (concatenate)(string[] ["OK", "ALL"] ("array"), w249) -> (w248:string[])
            n191 = Build Array (concatenate)(string[] ["OK", "ALL"] ("array"), w240) -> (w241:string[])
            n192 = property on="PLC" class="Ring (strict)"("Strings []"=w248, "Value"=1, "RingText.BGColor"=u32 16777088) -> ()  [unwired: 2 in, 2 out]
            n193 = property on="DB" class="Ring (strict)"("Strings []"=w241, "Value"=1, "RingText.BGColor"=u32 16777088) -> ()  [unwired: 2 in, 2 out]
          }
          frame #3 {
            # "Set default states before translation"
            n194 = Unbundle By Name(T12 {"Msg"=enum."Initializing", "Arguments"=[], "BgColor"=16744448, "TxtColor"=16448250, "Blink"=FALSE} ("UsrMsg")) -> ("BgColor"=w265:u32, "TxtColor"=w264:u32, "Blink"=w263:bool, "Msg"=w262:T6, "Arguments"=w261:variant[])
            n195 = call "Translator.Translate.Status (NoError).vi"("Arguments"=w261, "msg"=w262) -> ("Translated Msg"=w260:string)  [unwired: 9 in]
            n196 = property on="StatusMsg" class="Str"("Text.BGColor"=w265, "Text.TextColor"=w264, "Blinking"=w263, "Value"=w260) -> ()  [unwired: 2 in, 2 out]
          }
          frame #4 {
            # "Init Top Bar"
            n197 = global read "ApplicationGlobal.vi" "AppName-PC"() -> (w269:string)
            n198 = global read "ApplicationGlobal.vi" "AppVer-PC"() -> (w270:string)
            n199 = Format Into String(format string="%s %s", w269, w270) -> (resulting string=w271:string)  [unwired: 2 in, 1 out]
            n200 = global read "Config.Global.vi" "Touchpanel"() -> (w274:bool)
            n201 = local write "LogsOptions"(T2 {"IncludeBegin"=FALSE, "dtm_Begin"=timestamp(0 s since 1904-01-01), "IncludeEnd"=FALSE, "dtm_End"=timestamp(3588271200 s since 1904-01-01), "Events Level Operator"=enum.">=", "Level"=0, "Source"=0, "SearchText"="", "Refresh"=FALSE, "Pages"=0, "PageNo"=0, "First"=FALSE, "Prev"=FALSE, "Next"=FALSE, "Last"=FALSE} ("LogsOptions")) -> ()
            n202 = local read "TopBar"() -> (w268:T4)
            n203 = Bundle By Name(cluster=w268, "~touchpanel"=w274, "ver"=w271) -> (w273:T4)
            n204 = local write "TopBar"(w273) -> ()
          }
          frame #5 {
            w276 = T7."Disabled and Grayed Out" ("Disabled")
            n205 = property on="op20" class="Bool"("DisabledEnum"=w276) -> ()  [unwired: 2 in, 2 out]
            n206 = property on="op30_1" class="Bool"("DisabledEnum"=w276) -> ()  [unwired: 2 in, 2 out]
            n207 = property on="op10" class="Bool"("DisabledEnum"=w276) -> ()  [unwired: 2 in, 2 out]
            n208 = property on="check" class="Bool"("DisabledEnum"=T7."Enabled" ("Disabled")) -> ()  [unwired: 2 in, 2 out]
            n209 = property on="op40" class="Bool"("DisabledEnum"=w276) -> ()  [unwired: 2 in, 2 out]
            n210 = property on="op30_2" class="Bool"("DisabledEnum"=w276) -> ()  [unwired: 2 in, 2 out]
            n211 = property on="TESTER" class="Bool"("DisabledEnum"=w276) -> ()  [unwired: 2 in, 2 out]
          }
          frame #6 {
            (unwired) ""
            n212 = global read "Translator.Global.vi" "Flag"() -> (w283:picture)
            n213 = property on="Btn_Monitor" class="Bool (strict)"("Val(Sgnl)"=TRUE ("Value (Signaling)")) -> ()  [unwired: 2 in, 2 out]
            n214 = property on="~flag" class="Pict"("Value"=w283) -> ()  [unwired: 2 in, 2 out]
            n215 = property on="LogsMode" class="Enum (strict)"("Val(Sgnl)"=enum16{"Live", "Arch"}."Live" ("LogsMode")) -> ()  [unwired: 2 in, 2 out]
            n216 = property on="LogsTable" class="MCListbox (strict)"("ItemNames"=string[][] [] ("Item Names"), "TopLeft"=T8 {"Row"=0, "Column"=0} ("Top Left Visible Cell")) -> ()  [unwired: 2 in, 2 out]
            "LogsTable" <- -1 ("LogsTable")
          }
        }
      }
      frame "destructor" {
        # "Application shutdown actions"
        n217 = stacked-sequence {
          tunnel: w285 -> [_ _ _ _ w306 w307 _]
          tunnel: [_ _ _ _ _ w307 _] -> w284
          frame #0 {
            w295 = T9 {"Row"=-1, "Column"=-2} ("Active Cell:Active Cell")
            # "Restore controls to default state"
            # "Set default states before translation"
            n218 = call "Translator.Translate.Status (NoError).vi"("msg"=Translator.Message."Quitting") -> ("Translated Msg"=w302:string)  [unwired: 10 in]
            n219 = call "Wait.Gui.Open.vi"("Msg"=w302) -> ()  [unwired: 10 in, 1 out]
            n220 = property on="Btn_Exit" class="Bool (strict)"("Value"=FALSE ("Btn_Exit")) -> ()  [unwired: 2 in, 2 out]
            n221 = property on="StatusTable" class="MCListbox (strict)"("ActiveCell"=w295) -> (error out=w293:errorcluster, "CellBG"=w294:u32)  [unwired: 2 in, 1 out]
            n222 = property on="ErrMsg" class="MCListbox (strict)"("ItemNames"=string[][] [] ("Item Names"), "EditPos"=T9 {"Row"=-2, "Column"=-2} ("Edit Position"), "SelColor"=u32 16777216, "TopLeft"=T8 {"Row"=0, "Column"=0} ("Top Left Visible Cell"), "ActiveCell"=T9 {"Row"=-2, "Column"=-2} ("Active Cell:Active Cell"), "CellBG"=u32 13816530) -> ()  [unwired: 2 in, 2 out]
            n223 = property on="StatusTable" class="MCListbox (strict)"(error in=w293, "ActiveCell"=T9 {"Row"=-2, "Column"=-2} ("Active Cell:Active Cell"), "CellBG"=u32 16448250, "ActiveCell"=w295, "CellBG"=w294, "NumRows"=25, "TopLeft"=T8 {"Row"=0, "Column"=0} ("Top Left Visible Cell"), "ItemNames"=string[][] [] ("Item Names"), "Value"=-1 ("StatusTable")) -> ()  [unwired: 1 in, 2 out]
          }
          frame #1 {
          }
          frame #2 {
            # "Close references"
            n224 = local read "DeviceID"() -> (w304:refnum<k1>)
            n225 = call-poly <vilib>:"Close Input Device.vi"("device ID"=w304) -> ()  [unwired: 9 in, 1 out]
          }
          frame #3 {
            # "Close driver loops"
            n226 = call "PLC-Close.vi"("Idx"=0) -> ()  [unwired: 10 in, 1 out]
          }
          frame #4 {
            # "close database loops"
            n227 = call "Database-Kill.vi"("error in"=w306) -> ()  [unwired: 10 in, 1 out]
          }
          frame #5 {
            # "Translate VI back to English"
            n228 = call "Empty Picture"() -> ("empty picture"=w308:picture)
            n229 = property on="~flag" class="Pict"("Value"=w308) -> ()  [unwired: 2 in, 2 out]
          }
          frame #6 {
            # "Close all other loops"
            n230 = global write "User.Global.vi" "Guru"(FALSE ("Guru")) -> ()
            n231 = global write "User.Global.vi" "UserLoggedIn"(-1 ("UserLoggedIn")) -> ()
            n232 = global write "User.Global.vi" "UserLevel"(User.Level."-" ("UserLevel")) -> ()
            n233 = call "citTemplate.writeQueue.vi"("High priority (F)"=TRUE, "data in"="destructor") -> ()  [unwired: 13 in, 1 out]
          }
        }
      }
      frame "--- MainGui ---" {
        # "--> Handle error here..."
        # "Error handler"
        n234 = Unflatten From String(type=T14 {"ts"=timestamp(0 s since 1904-01-01), "src"=enum."All", "instance"=0, "action"="", "error"={"status"=FALSE, "code"=0, "source"=""}, "unconfirmed"=FALSE} ("ErrData"), binary string=w315, error in (no error)=w317) -> (error out=w314:errorcluster)  [unwired: 4 out]
      }
      frame "Gui.Translate" {
        n235 = global read "Translator.Global.vi" "Translations.Source"() -> (w321:string[])
        n236 = global read "Translator.Global.vi" "Translations.Level"() -> (w320:string[])
        n237 = property on="Level" class="Ring (strict)"("Strings []"=w320) -> ()  [unwired: 2 in, 2 out]
        n238 = property on="Source" class="Ring (strict)"("Strings []"=w321) -> ()  [unwired: 2 in, 2 out]
        n239 = call "MainGui-Error.vi"("error in (no error)"=w319) -> ("error out"=w318:errorcluster)  [unwired: 10 in]
        n240 = call "MainGui-StatusMsgUpdate.vi"("error in (no error)"=w318) -> ("error out"=w322:errorcluster)  [unwired: 10 in]
      }
      frame "Error.Update" {
        n241 = stacked-sequence {
          tunnel: w323 -> [w339 _]
          tunnel: [w336 _] -> w324
          frame #0 {
            n242 = call "ErrorHandling.Fglb.Get.vi"("error in (no error)"=w339) -> ("error out"=w337:errorcluster, "Errors"=w330:T14[], "unconfirmed?"=w333:bool)  [unwired: 8 in]
            n243 = for {
              tunnel: w330 -> [w357] mode=indexing
              tunnel: [w352] -> w338 mode=indexing
              n244 = Unbundle By Name(w357) -> ("src"=w346:T15, "ts"=w356:timestamp, "error.code"=w349:i32, "action"=w344:string, "error.source"=w350:string)
              n245 = Concatenate Strings(w344, " >> ", w350) -> (w345:string)
              n246 = Format Into String(format string="x%X", w349) -> (resulting string=w348:string)  [unwired: 2 in, 1 out]
              n247 = Format Into String(w346) -> (resulting string=w353:string)  [unwired: 3 in, 1 out]
              n248 = call "EventLog.FormatErrorMessage.vi"("Error string in"=w345) -> ("Error string out"=w351:string)
              n249 = Format Date/Time String(time format string (%c)="%H:%M:%S", seconds (now)=w356) -> (date/time string=w354:string)  [unwired: 1 in]
              n250 = Build Array(w353, w354, w348, w351) -> (w352:string[])
            }
            n251 = global write "ApplicationGlobal.vi" "UnconfirmedError"(w333) -> ()
            n252 = Empty Array?(array=w330) -> (empty?=w329:bool)
            n253 = Select(t=T7."Disabled and Grayed Out" ("Disabled"), s=w329, f=T7."Enabled" ("Disabled")) -> (s? t:f=w326:T7)
            n254 = property on="Btn_ErrConfirm" class="Bool"("DisabledEnum"=w326) -> ()  [unwired: 2 in, 2 out]
            n255 = Select(t=u32 16744576, s=w333, f=u32 13816530) -> (s? t:f=w331:u32)
            n256 = property on="ErrMsg" class="MCListbox (strict)"(error in=w337, "ItemNames"=w338, "DisabledEnum"=w326, "Value"=-1 ("ErrMsg"), "EditPos"=T9 {"Row"=-2, "Column"=-2} ("Edit Position"), "TopLeft"=T8 {"Row"=0, "Column"=0} ("Top Left Visible Cell"), "ActiveCell"=T9 {"Row"=-2, "Column"=-2} ("Active Cell:Active Cell"), "CellBG"=w331) -> (error out=w336:errorcluster)  [unwired: 1 in, 1 out]
            "ErrMsg" <- -1 ("ErrMsg")
          }
          frame #1 {
            n257 = control-ref of="ErrMsg"() -> (w358:refnum<vi>)
            n258 = call "Table.AutoSize.vi"("Table"=w358) -> ()  [unwired: 11 in]
          }
        }
      }
      frame "Error.Confirm" {
        n259 = call "ErrorHandling.Fglb.Confirm.vi"("error in (no error)"=w360) -> ("error out"=w359:errorcluster)  [unwired: 10 in]
      }
      frame "TopBar.Update" {
        n260 = stacked-sequence {
          frame #0 {
            w362 = u64 0 ("Reference")
            n261 = Greater Than 0?(x=w362) -> (x > 0?=w372:bool)
            n262 = call "RefNumFormat.vi"("RefNum Val"=w362) -> ("RefNum String"=w371:string)  [unwired: 1 out]
            n263 = Select(t=w371, s=w372, f="") -> (s? t:f=w368:string)
            n264 = Format Date/Time String(time format string (%c)="%Y-%m-%d %H:%M:%S") -> (date/time string=w366:string)  [unwired: 2 in]
            n265 = call <vilib>:"Trim Whitespace.vi"("string"=w368) -> ("trimmed string"=w369:string)  [unwired: 1 in]
            n266 = Bundle By Name(cluster="TopBar", "time"=w366, "~msg"=w369) -> (w364:T4)
            n267 = Unbundle By Name(w364) -> ("~touchpanel"=w365:T5)
            n268 = local write "TopBar"(w364) -> ()
            n269 = global write "Config.Global.vi" "Touchpanel"(w365) -> ()
          }
          frame #1 {
            n270 = global read "Database.Global.vi" "DB.Status"() -> (w383:T22)
            n271 = global read "Database.Global.vi" "DB.Sets"() -> (w381:T23)
            n272 = Unbundle By Name(w381) -> ("Enable"=w382:bool)
            n273 = Unbundle By Name(w383) -> ("Run"=w374:bool)
            n274 = Build Array(w382) -> (w373:bool[])
            n275 = Build Array(w374) -> (w380:bool[])
            n276 = Compound Arithmetic op=OR(invert w373, w380) -> (w384:bool[])
            n277 = Search 1D Array(1D array=w384, element=FALSE) -> (index of element=w386:i32)  [unwired: 1 in]
            n278 = Increment(x=w386) -> (x+1=w375:i32)
            n279 = Less Or Equal To 0?(x=w375) -> (x <= 0?=w377:bool)
            n280 = Select(t=u32 8454016, s=w377, f=u32 16744576) -> (s? t:f=w376:u32)
            n281 = property on="DB" class="Ring (strict)"("Value"=w375, "RingText.BGColor"=w376) -> ()  [unwired: 2 in, 2 out]
          }
          frame #2 {
            n282 = global read "PLC.Global.vi" "PLC1.Status"() -> (w400:T21)
            n283 = global read "PLC.Global.vi" "PLC1.Sets"() -> (w399:T24)
            n284 = Build Array(w400) -> (w398:T21[])
            n285 = Build Array(w399) -> (w397:T24[])
            n286 = for {
              tunnel: w398 -> [w407] mode=indexing
              tunnel: [w405] -> w390 mode=indexing
              tunnel: w397 -> [w406] mode=indexing
              n287 = Unbundle By Name(w407) -> ("State"=w403:T16)
              n288 = Unbundle By Name(w406) -> ("Enable"=w404:bool)
              n289 = Greater Or Equal?(x=w403, y=PLC.State."Idle" ("State")) -> (x >= y?=w402:bool)
              n290 = Compound Arithmetic op=OR(w402, invert w404) -> (w405:bool)
            }
            n291 = And Array Elements(Boolean array=w390) -> (logical AND=w391:bool)
            n292 = Build Array (concatenate)(w391, w390) -> (w389:bool[])
            n293 = Search 1D Array(1D array=w389, element=FALSE) -> (index of element=w394:i32)  [unwired: 1 in]
            n294 = Increment(x=w394) -> (x+1=w387:i32)
            n295 = Less Or Equal To 0?(x=w387) -> (x <= 0?=w388:bool)
            n296 = Select(t=u32 8454016, s=w388, f=u32 16744576) -> (s? t:f=w392:u32)
            n297 = property on="PLC" class="Ring (strict)"("Value"=w387, "RingText.BGColor"=w392) -> ()  [unwired: 2 in, 2 out]
          }
        }
      }
      frame "Buttons.Update" {
        n298 = global read "ApplicationGlobal.vi" "Unlock"() -> (w408:bool)
        n299 = local write "Btin_LogIn"(w408) -> ()
      }
      frame "StatusMsg.Update" {
        # "Update status of running sequence"
        n300 = property on="DB" class="Ring (strict)"() -> ("Value"=w417:u16)  [unwired: 2 in, 2 out]
        n301 = property on="PLC" class="Ring (strict)"() -> ("Value"=w416:u16)  [unwired: 2 in, 2 out]
        n302 = Greater Than 0?(x=w416) -> (x > 0?=w415:bool)
        n303 = Greater Than 0?(x=w417) -> (x > 0?=w414:bool)
        n304 = Compound Arithmetic op=OR(w415, w414) -> (w411:bool)
        n305 = feedback-in #1(w411) -> ()
        n306 = feedback #1() -> (w410:bool)  [unwired: 1 in]
        n307 = case shown="False" w411 {
          selector: w411 -> [_ w432]
          tunnel: w414 -> [w429 _]
          tunnel: w413 -> [w419 w434]
          tunnel: [w418 w433] -> w412
          tunnel: w410 -> [_ w431]
          frame True {
            (unwired) T12 {"Msg"=enum."Reconnecting DB", "Arguments"=[], "BgColor"=16744576, "TxtColor"=0, "Blink"=FALSE} ("UsrMsg")
            (unwired) T12 {"Msg"=enum."Reconnecting DB", "Arguments"=[], "BgColor"=16744576, "TxtColor"=0, "Blink"=FALSE} ("UsrMsg")
            (unwired) T12 {"Msg"=enum."Reconnecting DB", "Arguments"=[], "BgColor"=16744576, "TxtColor"=0, "Blink"=FALSE} ("UsrMsg")
            n308 = Select(t=T12 {"Msg"=enum."Reconnecting DB", "Arguments"=[], "BgColor"=16744576, "TxtColor"=0, "Blink"=FALSE} ("UsrMsg"), s=w429, f=T12 {"Msg"=enum."Reconnecting PLC", "Arguments"=[], "BgColor"=16744576, "TxtColor"=0, "Blink"=FALSE} ("UsrMsg")) -> (s? t:f=w420:T12)
            n309 = Unbundle By Name(w420) -> ("BgColor"=w421:u32, "TxtColor"=w422:u32, "Blink"=w423:bool, "Msg"=w424:T6, "Arguments"=w426:variant[])
            n310 = call "Translator.Translate.Status (NoError).vi"("Arguments"=w426, "msg"=w424) -> ("Translated Msg"=w425:string)  [unwired: 9 in]
            n311 = property on="StatusMsg" class="Str"(error in=w419, "Text.BGColor"=w421, "Text.TextColor"=w422, "Blinking"=w423, "Value"=w425) -> (error out=w418:errorcluster)  [unwired: 1 in, 1 out]
          }
          frame False {
            n312 = Not Equal?(x=w431, y=w432) -> (x != y?=w430:bool)
            n313 = case shown="True" w430 {
              tunnel: w434 -> [w435 w438]
              tunnel: [w435 w437] -> w433
              frame False {
              }
              frame True {
                n314 = Unbundle By Name(T12 {"Msg"=enum."IDLE", "Arguments"=[], "BgColor"=13816530, "TxtColor"=0, "Blink"=FALSE} ("UsrMsg")) -> ("BgColor"=w439:u32, "TxtColor"=w440:u32, "Blink"=w441:bool, "Msg"=w442:T6, "Arguments"=w444:variant[])
                n315 = call "Translator.Translate.Status (NoError).vi"("Arguments"=w444, "msg"=w442) -> ("Translated Msg"=w443:string)  [unwired: 9 in]
                n316 = property on="StatusMsg" class="Str"(error in=w438, "Text.BGColor"=w439, "Text.TextColor"=w440, "Blinking"=w441, "Value"=w443) -> (error out=w437:errorcluster)  [unwired: 1 in, 1 out]
              }
            }
          }
        }
      }
      frame "StatusTable.Update" {
        n317 = control-ref of="This VI"() -> (w453:refnum<vi>)
        n318 = Unflatten From String(type=T17 {"Station"="", "ButtonEnabled"=FALSE, "Values"=[]} ("TestValueResult"), binary string=w458, error in (no error)=w460) -> (value=w457:T17, error out=w451:errorcluster)  [unwired: 2 in, 1 out]
        n319 = property class="VI"(reference=w453) -> ("Panel"=w452:refnum<vi>)  [unwired: 1 in, 2 out]
        n320 = property class="Pnl"(reference=w452, "DeferPanUpdts"=TRUE) -> (reference out=w447:refnum<vi>, error out=w450:errorcluster)  [unwired: 1 in]
        n321 = Unbundle By Name(w457) -> ("Station"=w454:string, "ButtonEnabled"=w456:bool, "Values"=w455:T18[])
        n322 = Merge Errors(w451, w450) -> (w445:errorcluster)
        n323 = case shown="\"OP10\"" w454 {
          tunnel: w456 -> [_ w494 w497 w501 w505 w509 w512]
          frame Default {
          }
          frame "OP10" {
            w492 = T7."Enabled" ("Disabled")
            n324 = Select(t=w492, s=w494, f=T7."Disabled and Grayed Out" ("Disabled")) -> (s? t:f=w493:T7)
            n325 = property on="op10" class="Bool"("DisabledEnum"=w492) -> ()  [unwired: 2 in, 2 out]
            n326 = property on="op20" class="Bool"("DisabledEnum"=w493) -> ()  [unwired: 2 in, 2 out]
          }
          frame "OP20" {
            n327 = Select(t=T7."Enabled" ("Disabled"), s=w497, f=T7."Disabled and Grayed Out" ("Disabled")) -> (s? t:f=w496:T7)
            n328 = property on="op30_1" class="Bool"("DisabledEnum"=w496) -> ()  [unwired: 2 in, 2 out]
          }
          frame "OP30_1" {
            n329 = Select(t=T7."Enabled" ("Disabled"), s=w501, f=T7."Disabled and Grayed Out" ("Disabled")) -> (s? t:f=w500:T7)
            n330 = property on="op30_2" class="Bool"("DisabledEnum"=w500) -> ()  [unwired: 2 in, 2 out]
          }
          frame "OP30_2" {
            n331 = Select(t=T7."Enabled" ("Disabled"), s=w505, f=T7."Disabled and Grayed Out" ("Disabled")) -> (s? t:f=w504:T7)
            n332 = property on="TESTER" class="Bool"("DisabledEnum"=w504) -> ()  [unwired: 2 in, 2 out]
          }
          frame "TESTER" {
            n333 = Select(t=T7."Enabled" ("Disabled"), s=w509, f=T7."Disabled and Grayed Out" ("Disabled")) -> (s? t:f=w508:T7)
            n334 = property on="op40" class="Bool"("DisabledEnum"=w508) -> ()  [unwired: 2 in, 2 out]
          }
          frame "OP40" {
            n335 = Select(t=T7."Enabled" ("Disabled"), s=w512, f=T7."Disabled and Grayed Out" ("Disabled")) -> (s? t:f=w513:T7)
            n336 = property on="op40" class="Bool"("DisabledEnum"=w513) -> ()  [unwired: 2 in, 2 out]
          }
        }
        n337 = for {
          tunnel: w455 -> [w481] mode=indexing
          tunnel: w454 -> [w480]
          tunnel: w445 -> [_]
          tunnel: [w461] -> w446
          w462 = "%.5f" ("format string")
          n338 = Unbundle By Name(w481) -> ("EV_name"=w479:string, "Status"=w464:u8, "LimitL"=w466:dbl, "Value"=w473:dbl, "LimitH"=w467:dbl)
          n339 = property on="StatusTable" class="MCListbox (strict)"() -> ("ItemNames"=w470:string[][])  [unwired: 2 in, 2 out]
          n340 = Number To Decimal String(number=w464) -> (decimal integer string=w478:string)  [unwired: 1 in]
          n341 = Format Value(format string=w462, value (0)=w466) -> (output string=w477:string)  [unwired: 1 in]
          n342 = Format Value(format string=w462, value (0)=w473) -> (output string=w476:string)  [unwired: 1 in]
          n343 = Format Value(format string=w462, value (0)=w467) -> (output string=w475:string)  [unwired: 1 in]
          n344 = Build Array(w480, w479, w478, w477, w476, w475) -> (w474:string[])
          n345 = Build Array (concatenate)(w470, w474) -> (w469:string[][])
          n346 = Array Size(array=w469) -> (size(s)=w468:i32[])
          n347 = Index Array(array=w468) -> (element #1=w471:i32, element #2=w472:i32)  [unwired: 2 in]
          n348 = Equal?(x=w464, y=1) -> (x = y?=w463:bool)
          n349 = for {
            N: w472 -> [_]
            tunnel: w471 -> [w489]
            tunnel: w463 -> [w487]
            tunnel: [w482] -> w461
            i -> [w490]
            n350 = Decrement(x=w489) -> (x-1=w483:i32)
            n351 = Bundle By Name(cluster=T9 {"Row"=0, "Column"=0} ("Active Cell:Active Cell"), "Row"=w483, "Column"=w490) -> (w488:T9)
            n352 = Select(t=u32 6618880, s=w487, f=u32 16711680) -> (s? t:f=w484:u32)
            n353 = property on="StatusTable" class="MCListbox (strict)"("ActiveCell"=w488, "CellBG"=w484) -> (error out=w482:errorcluster)  [unwired: 2 in, 1 out]
          }
          n354 = property on="StatusTable" class="MCListbox (strict)"("ItemNames"=w469) -> ()  [unwired: 2 in, 2 out]
        }
        n355 = property class="Pnl"(reference=w447, error in=w446, "DeferPanUpdts"=FALSE) -> ()  [unwired: 2 out]
      }
      frame "LogsTable.Update" {
        n356 = stacked-sequence {
          tunnel: w517 -> [_ _ w526 _ _]
          tunnel: [_ _ w529 _ _] -> w516
          frame #0 {
            n357 = call "Panel.Disable.vi"("Defer Panel Updates (F)"=TRUE) -> ()  [unwired: 10 in, 1 out]
          }
          frame #1 {
          }
          frame #2 {
            n358 = local read "LogsMode"() -> (w519:enum16{"Live", "Arch"})
            n359 = global read "ApplicationGlobal.vi" "EventPath"() -> (w524:path)
            n360 = property on="LogsTable" class="MCListbox (strict)"() -> ("NumRows"=w525:u32)  [unwired: 2 in, 2 out]
            n361 = global read "Translator.Global.vi" "Translations.Source"() -> (w532:string[])
            n362 = global read "Translator.Global.vi" "Translations.Level"() -> (w530:string[])
            n363 = case shown="\"Live\"" w519 {
              tunnel: w526 -> [w536 w543]
              tunnel: w525 -> [_ w542]
              tunnel: w524 -> [_ w541]
              tunnel: "LogsOptions" -> [w533 w540]
              tunnel: [w535 w539] -> w522
              tunnel: [w534 w538] -> w521
              tunnel: [w533 w537] -> w520
              frame "Live" {
                n364 = call "EventLog.Buffer.vi"("error in"=w536, "Event.Sets"=w533) -> ("error out"=w535:errorcluster, "data out"=w534:T25[])  [unwired: 6 in, 2 out]
              }
              frame Default {
                n365 = call "EventLog.ListFiles.vi"("Sets in"=w540, "error in"=w543, "Size"=w542, "Path"=w541) -> ("error out"=w539:errorcluster, "Events"=w538:T25[], "Sets out"=w537:T2)  [unwired: 5 in]
              }
            }
            n366 = Format Date/Time String(time format string (%c)="%Y-%m-%d ") -> (date/time string=w527:string)  [unwired: 2 in]
            n367 = for {
              tunnel: [w563] -> w531 mode=indexing
              tunnel: w521 -> [w562] mode=indexing
              tunnel: w530 -> [w561]
              tunnel: w532 -> [w557]
              tunnel: w527 -> [w551]
              n368 = Unbundle By Name(w562) -> ("ts"=w554:dbl, "src"=w549:T15, "msg_str"=w560:string, "lev"=w559:T26)
              n369 = To Long Integer(number=w559) -> (32bit integer=w556:i32)
              n370 = Index Array(array=w557, index=w549) -> (element=w550:string)
              n371 = Increment(x=w556) -> (x+1=w558:i32)
              n372 = Format Date/Time String(time format string (%c)="%Y-%m-%d ", seconds (now)=w554) -> (date/time string=w548:string)  [unwired: 1 in]
              n373 = Format Date/Time String(time format string (%c)="%H:%M:%S%3u", seconds (now)=w554) -> (date/time string=w545:string)  [unwired: 1 in]
              n374 = Index Array(array=w561, index=w558) -> (element=w555:string)
              n375 = Not Equal?(x=w551, y=w548) -> (x != y?=w546:bool)
              n376 = Concatenate Strings(w548, w545) -> (w547:string)
              n377 = Select(t=w547, s=w546, f=w545) -> (s? t:f=w544:string)
              n378 = Build Array(w544, w555, w550, w560) -> (w563:string[])
            }
            n379 = local write "LogsOptions"(w520) -> ()
            n380 = property on="LogsTable" class="MCListbox (strict)"(error in=w522, "ItemNames"=w531) -> (error out=w529:errorcluster)  [unwired: 1 in, 1 out]
          }
          frame #3 {
            n381 = Get Date/Time In Seconds() -> (seconds since 1Jan1904=w566:timestamp)
            n382 = Add(x=w566, y=5.0) -> (x+y=→"RefreshDelay":timestamp)
            n383 = control-ref of="LogsTable"() -> (w567:refnum<vi>)
            n384 = call "Table.AutoSize.vi"("Table"=w567) -> ()  [unwired: 11 in]
          }
          frame #4 {
            n385 = call "Panel.Disable.vi"() -> ()  [unwired: 11 in, 1 out]
          }
        }
      }
      frame "PLCReasemblyDone" {
        n386 = local read "LastPlcRequest"() -> (w583:T1)
        n387 = Unflatten From String(type=w583, binary string=w568, error in (no error)=w587) -> (value=w584:T1, error out=w569:errorcluster)  [unwired: 2 in, 1 out]
        n388 = Equal?(x=w583, y=w584) -> (x = y?=w580:T27)
        n389 = Cluster To Array(cluster=w580) -> (array=w579:bool[])
        n390 = And Array Elements(Boolean array=w579) -> (logical AND=w574:bool)
        n391 = Select(t="Produkt %s | %s wrocil na stacjei%s", s=w574, f="Nie udalo sie powrocic produktem %s | %s na stacje%s") -> (s? t:f=w576:string)
        n392 = Select(t=u32 6618880, s=w574, f=u32 16711680) -> (s? t:f=w571:u32)
        n393 = Unbundle By Name(w583) -> ("Ref"=w586:string, "Serial"=w581:string, "Station"=w582:string)
        n394 = Format Into String(format string=w576, w586, w581, w582) -> (resulting string=w575:string)  [unwired: 2 in, 1 out]
        n395 = property on="StatusMsg" class="Str"("Text.BGColor"=w571, "Text.TextColor"=u32 0, "Value"=w575) -> ()  [unwired: 2 in, 2 out]
        n396 = flat-sequence {
          tunnel: w569 -> [_]
          frame #0 {
            n397 = local write "LastRequestedProduct"(cluster{"Variant":string, "Serial":string} {"Variant"="", "Serial"=""} ("LastRequestedProduct")) -> ()
            n398 = local write "LastPlcRequest"(T1 {"Ref"="", "Serial"="", "Station"=""} ("LastPlcRequest")) -> ()
          }
        }
        n399 = property on="check" class="Bool"("DisabledEnum"=T7."Enabled" ("Disabled")) -> ()  [unwired: 2 in, 2 out]
      }
    }
    n400 = call "citTemplate.ErrorEventPass.vi"("error in"=w2, "action of error"=w4, "event in"=w8) -> ("error out"=w5:errorcluster)  [unwired: 2 in, 6 out]
  }
